vi "SetTorqueWaveformUnit.vi"(8 "error in (no error)":errorcluster, 9 "Waveform in":waveform(sgl), 11 "Name":string) -> (0 "error out":errorcluster, 1 "Waveform out":waveform(sgl))   [LabVIEW 2017, in "McsaUtilities.lvlib"]
uses:
  <vilib>/addons/InsightCM/Utilities/MCSA/McsaUtilities.lvlib
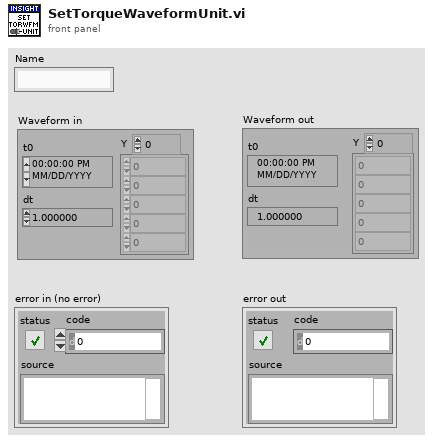
[diagram p1: front panel]
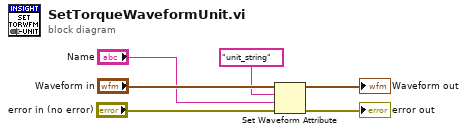
[diagram p0: block diagram]
diagram:
  n1 = Set Waveform Attribute(4:"error in (no error)", 5:"Name", 6:"unit_string" ("name"), 7:"Waveform in") -> (0:→"error out":errorcluster, 3:→"Waveform out":waveform(sgl))  [unwired: 1 out]
